vi "GeoData.vi"() -> ()   [LabVIEW 2017] (continued)
48213\tPalestine\tTX\tHenderson County\tH1\n75763\t48213\tFrankston\tTX\tHenderson County\tH1\n75778\t48213\tMurchison\tTX\tHenderson County\tH1\n75751\t48213\tAthens\tTX\tHenderson County\tH1\n75124\t48213\tEustace\tTX\tHenderson County\tH1\n75143\t48213\tKemp\tTX\tHenderson County\tH1\n75782\t48213\tPoynor\tTX\tHenderson County\tH1\n75148\t48213\tMalakoff\tTX\tHenderson County\tH1\n75758\t48213\tChandler\tTX\tHenderson County\tH1\n75147\t48213\tMabank\tTX\tHenderson County\tH1\n75163\t48213\tTrinidad\tTX\tHenderson County\tH1\n75752\t48213\tAthens\tTX\tHenderson County\tH1\n75770\t48213\tLarue\tTX\tHenderson County\tH1\n75756\t48213\tBrownsboro\tTX\tHenderson County\tH1\n75156\t48213\tMabank\tTX\tHenderson County\tH1\n78537\t48215\tDonna\tTX\tHidalgo County\tH1\n78573\t48215\tMission\tTX\tHidalgo County\tH1\n78569\t48215\tLyford\tTX\tHidalgo County\tH1\n78563\t48215\tLinn\tTX\tHidalgo County\tH1\n78502\t48215\tMcallen\tTX\tHidalgo County\tH1\n78501\t48215\tMcallen\tTX\tHidalgo County\tH1\n78599\t48215\tWeslaco\tTX\tHidalgo County\tH1\n78549\t48215\tHargill\tTX\tHidalgo County\tH1\n78504\t48215\tMcallen\tTX\tHidalgo County\tH1\n78516\t48215\tAlamo\tTX\tHidalgo County\tH1\n78538\t48215\tEdcouch\tTX\tHidalgo County\tH1\n78596\t48215\tWeslaco\tTX\tHidalgo County\tH1\n78505\t48215\tMcallen\tTX\tHidalgo County\tH1\n78548\t48215\tGrulla\tTX\tHidalgo County\tH1\n78562\t48215\tLa villa\tTX\tHidalgo County\tH1\n78540\t48215\tEdinburg\tTX\tHidalgo County\tH1\n78558\t48215\tLa blanca\tTX\tHidalgo County\tH1\n78577\t48215\tPharr\tTX\tHidalgo County\tH1\n78570\t48215\tMercedes\tTX\tHidalgo County\tH1\n78579\t48215\tProgreso\tTX\tHidalgo County\tH1\n78595\t48215\tSullivan city\tTX\tHidalgo County\tH1\n78503\t48215\tMcallen\tTX\tHidalgo County\tH1\n78541\t48215\tEdinburg\tTX\tHidalgo County\tH1\n78572\t48215\tMission\tTX\tHidalgo County\tH1\n78557\t48215\tHidalgo\tTX\tHidalgo County\tH1\n78559\t48215\tLa feria\tTX\tHidalgo County\tH1\n78539\t48215\tEdinburg\tTX\tHidalgo County\tH1\n78542\t48215\tEdinburg\tTX\tHidalgo County\tH1\n78574\t48215\tMission\tTX\tHidalgo County\tH1\n78576\t48215\tPenitas\tTX\tHidalgo County\tH1\n78589\t48215\tSan juan\tTX\tHidalgo County\tH1\n78560\t48215\tLa joya\tTX\tHidalgo County\tH1\n78543\t48215\tElsa\tTX\tHidalgo County\tH1\n78565\t48215\tLos ebanos\tTX\tHidalgo County\tH1\n76055\t48217\tItasca\tTX\tHill County\tH1\n76692\t48217\tWhitney\tTX\tHill County\tH1\n76627\t48217\tBlum\tTX\tHill County\tH1\n76622\t48217\tAquilla\tTX\tHill County\tH1\n76093\t48217\tRio vista\tTX\tHill County\tH1\n76676\t48217\tPenelope\tTX\tHill County\tH1\n76628\t48217\tBrandon\tTX\tHill County\tH1\n76621\t48217\tAbbott\tTX\tHill County\tH1\n76631\t48217\tBynum\tTX\tHill County\tH1\n76650\t48217\tIrene\tTX\tHill County\tH1\n76050\t48217\tGrandview\tTX\tHill County\tH1\n76691\t48217\tWest\tTX\tHill County\tH1\n76648\t48217\tHubbard\tTX\tHill County\tH1\n76636\t48217\tCovington\tTX\tHill County\tH1\n76670\t48217\tMilford\tTX\tHill County\tH1\n76645\t48217\tHillsboro\tTX\tHill County\tH1\n76673\t48217\tMount calm\tTX\tHill County\tH1\n76660\t48217\tMalone\tTX\tHill County\tH1\n76666\t48217\tMertens\tTX\tHill County\tH1\n79358\t48219\tRopesville\tTX\tHockley County\tH1\n79407\t48219\tLubbock\tTX\tHockley County\tH1\n79363\t48219\tShallowater\tTX\tHockley County\tH1\n79313\t48219\tAnton\tTX\tHockley County\tH1\n79372\t48219\tSundown\tTX\tHockley County\tH1\n79345\t48219\tMeadow\tTX\tHockley County\tH1\n79367\t48219\tSmyer\tTX\tHockley County\tH1\n79380\t48219\tWhitharral\tTX\tHockley County\tH1\n79339\t48219\tLittlefield\tTX\tHockley County\tH1\n79336\t48219\tLevelland\tTX\tHockley County\tH1\n79353\t48219\tPep\tTX\tHockley County\tH1\n76035\t48221\tCresson\tTX\tHood County\tH1\n76462\t48221\tLipan\tTX\tHood County\tH1\n76048\t48221\tGranbury\tTX\tHood County\tH1\n76033\t48221\tCleburne\tTX\tHood County\tH1\n76049\t48221\tGranbury\tTX\tHood County\tH1\n76433\t48221\tBluff dale\tTX\tHood County\tH1\n76476\t48221\tTolar\tTX\tHood County\tH1\n76087\t48221\tWeatherford\tTX\tHood County\tH1\n76044\t48221\tGodley\tTX\tHood County\tH1\n76467\t48221\tPaluxy\tTX\tHood County\tH1\n75431\t48223\tComo\tTX\tHopkins County\tH1\n75457\t48223\tMount vernon\tTX\tHopkins County\tH1\n75420\t48223\tBrashear\tTX\tHopkins County\tH1\n75497\t48223\tYantis\tTX\tHopkins County\tH1\n75481\t48223\tSulphur bluff\tTX\tHopkins County\tH1\n75453\t48223\tLone oak\tTX\tHopkins County\tH1\n75494\t48223\tWinnsboro\tTX\tHopkins County\tH1\n75437\t48223\tDike\tTX\tHopkins County\tH1\n75482\t48223\tSulphur springs\tTX\tHopkins County\tH1\n75471\t48223\tPickton\tTX\tHopkins County\tH1\n75483\t48223\tSulphur springs\tTX\tHopkins County\tH1\n75433\t48223\tCumby\tTX\tHopkins County\tH1\n75478\t48223\tSaltillo\tTX\tHopkins County\tH1\n75862\t48225\tTrinity\tTX\tHouston County\tH1\n75844\t48225\tGrapeland\tTX\tHouston County\tH1\n75849\t48225\tLatexo\tTX\tHouston County\tH1\n75847\t48225\tKennard\tTX\tHouston County\tH1\n75839\t48225\tElkhart\tTX\tHouston County\tH1\n75858\t48225\tRatcliff\tTX\tHouston County\tH1\n75851\t48225\tLovelady\tTX\tHouston County\tH1\n75835\t48225\tCrockett\tTX\tHouston County\tH1\n79511\t48227\tCoahoma\tTX\tHoward County\tH1\n79720\t48227\tBig spring\tTX\tHoward County\tH1\n79733\t48227\tForsan\tTX\tHoward County\tH1\n79748\t48227\tKnott\tTX\tHoward County\tH1\n79851\t48229\tSierra blanca\tTX\tHudspeth County\tH1\n79837\t48229\tDell city\tTX\tHudspeth County\tH1\n79839\t48229\tFort hancock\tTX\tHudspeth County\tH1\n79938\t48229\tEl paso\tTX\tHudspeth County\tH1\n75474\t48231\tQuinlan\tTX\tHunt County\tH1\n75469\t48231\tPecan gap\tTX\tHunt County\tH1\n75402\t48231\tGreenville\tTX\tHunt County\tH1\n75423\t48231\tCeleste\tTX\tHunt County\tH1\n75169\t48231\tWills point\tTX\tHunt County\tH1\n75442\t48231\tFarmersville\tTX\tHunt County\tH1\n75428\t48231\tCommerce\tTX\tHunt County\tH1\n75422\t48231\tCampbell\tTX\tHunt County\tH1\n75160\t48231\tTerrell\tTX\tHunt County\tH1\n75448\t48231\tKlondike\tTX\tHunt County\tH1\n75401\t48231\tGreenville\tTX\tHunt County\tH1\n75453\t48231\tLone oak\tTX\tHunt County\tH1\n75403\t48231\tGreenville\tTX\tHunt County\tH1\n75496\t48231\tWolfe city\tTX\tHunt County\tH1\n75135\t48231\tCaddo mills\tTX\tHunt County\tH1\n75452\t48231\tLeonard\tTX\tHunt County\tH1\n75449\t48231\tLadonia\tTX\tHunt County\tH1\n75458\t48231\tMerit\tTX\tHunt County\tH1\n75189\t48231\tRoyse city\tTX\tHunt County\tH1\n75404\t48231\tGreenville\tTX\tHunt County\tH1\n79080\t48233\tSkellytown\tTX\tHutchinson County\tH1\n79078\t48233\tSanford\tTX\tHutchinson County\tH1\n79036\t48233\tFritch\tTX\tHutchinson County\tH1\n79008\t48233\tBorger\tTX\tHutchinson County\tH1\n79062\t48233\tMorse\tTX\tHutchinson County\tH1\n79081\t48233\tSpearman\tTX\tHutchinson County\tH1\n79083\t48233\tStinnett\tTX\tHutchinson County\tH1\n79007\t48233\tBorger\tTX\tHutchinson County\tH1\n76941\t48235\tMertzon\tTX\tIrion County\tH1\n76904\t48235\tSan angelo\tTX\tIrion County\tH1\n76901\t48235\tSan angelo\tTX\tIrion County\tH1\n76930\t48235\tBarnhart\tTX\tIrion County\tH1\n76449\t48237\tGraford\tTX\tJack County\tH1\n76459\t48237\tJermyn\tTX\tJack County\tH1\n76487\t48237\tPoolville\tTX\tJack County\tH1\n76486\t48237\tPerrin\tTX\tJack County\tH1\n76426\t48237\tBridgeport\tTX\tJack County\tH1\n76365\t48237\tHenrietta\tTX\tJack County\tH1\n76431\t48237\tChico\tTX\tJack County\tH1\n76427\t48237\tBryson\tTX\tJack County\tH1\n76230\t48237\tBowie\tTX\tJack County\tH1\n76389\t48237\tWindthorst\tTX\tJack County\tH1\n76458\t48237\tJacksboro\tTX\tJack County\tH1\n77979\t48239\tPort lavaca\tTX\tJackson County\tH1\n77957\t48239\tEdna\tTX\tJackson County\tH1\n77465\t48239\tPalacios\tTX\tJackson County\tH1\n77971\t48239\tLolita\tTX\tJackson County\tH1\n77969\t48239\tLa salle\tTX\tJackson County\tH1\n77962\t48239\tGanado\tTX\tJackson County\tH1\n77991\t48239\tVanderbilt\tTX\tJackson County\tH1\n77961\t48239\tFrancitas\tTX\tJackson County\tH1\n77970\t48239\tLa ward\tTX\tJackson County\tH1\n75933\t48241\tCall\tTX\tJasper County\tH1\n75966\t48241\tNewton\tTX\tJasper County\tH1\n77662\t48241\tVidor\tTX\tJasper County\tH1\n75931\t48241\tBrookeland\tTX\tJasper County\tH1\n75951\t48241\tJasper\tTX\tJasper County\tH1\n75980\t48241\tZavalla\tTX\tJasper County\tH1\n75956\t48241\tKirbyville\tTX\tJasper County\tH1\n77615\t48241\tEvadale\tTX\tJasper County\tH1\n77612\t48241\tBuna\tTX\tJasper County\tH1\n79734\t48243\tFort davis\tTX\tJeff Davis County\tH1\n79854\t48243\tValentine\tTX\tJeff Davis County\tH1\n77702\t48245\tBeaumont\tTX\tJefferson County\tH1\n77622\t48245\tHamshire\tTX\tJefferson County\tH1\n77726\t48245\tBeaumont\tTX\tJefferson County\tH1\n77707\t48245\tBeaumont\tTX\tJefferson County\tH1\n77705\t48245\tBeaumont\tTX\tJefferson County\tH1\n77651\t48245\tPort neches\tTX\tJefferson County\tH1\n77613\t48245\tChina\tTX\tJefferson County\tH1\n77665\t48245\tWinnie\tTX\tJefferson County\tH1\n77619\t48245\tGroves\tTX\tJefferson County\tH1\n77655\t48245\tSabine pass\tTX\tJefferson County\tH1\n77629\t48245\tNome\tTX\tJefferson County\tH1\n77706\t48245\tBeaumont\tTX\tJefferson County\tH1\n77720\t48245\tBeaumont\tTX\tJefferson County\tH1\n77725\t48245\tBeaumont\tTX\tJefferson County\tH1\n77642\t48245\tPort arthur\tTX\tJefferson County\tH1\n77657\t48245\tLumberton\tTX\tJefferson County\tH1\n77701\t48245\tBeaumont\tTX\tJefferson County\tH1\n77704\t48245\tBeaumont\tTX\tJefferson County\tH1\n77708\t48245\tBeaumont\tTX\tJefferson County\tH1\n77713\t48245\tBeaumont\tTX\tJefferson County\tH1\n77627\t48245\tNederland\tTX\tJefferson County\tH1\n77640\t48245\tPort arthur\tTX\tJefferson County\tH1\n77703\t48245\tBeaumont\tTX\tJefferson County\tH1\n78582\t48247\tRio grande city\tTX\tJim Hogg County\tH1\n78360\t48247\tGuerra\tTX\tJim Hogg County\tH1\n78361\t48247\tHebbronville\tTX\tJim Hogg County\tH1\n78383\t48249\tSandia\tTX\tJim Wells County\tH1\n78372\t48249\tOrange grove\tTX\tJim Wells County\tH1\n78375\t48249\tPremont\tTX\tJim Wells County\tH1\n78384\t48249\tSan diego\tTX\tJim Wells County\tH1\n78342\t48249\tBen bolt\tTX\tJim Wells County\tH1\n78332\t48249\tAlice\tTX\tJim Wells County\tH1\n78380\t48249\tRobstown\tTX\tJim Wells County\tH1\n76059\t48251\tKeene\tTX\tJohnson County\tH1\n76035\t48251\tCresson\tTX\tJohnson County\tH1\n76084\t48251\tVenus\tTX\tJohnson County\tH1\n76033\t48251\tCleburne\tTX\tJohnson County\tH1\n76093\t48251\tRio vista\tTX\tJohnson County\tH1\n76009\t48251\tAlvarado\tTX\tJohnson County\tH1\n76061\t48251\tLillian\tTX\tJohnson County\tH1\n76058\t48251\tJoshua\tTX\tJohnson County\tH1\n76049\t48251\tGranbury\tTX\tJohnson County\tH1\n76050\t48251\tGrandview\tTX\tJohnson County\tH1\n76036\t48251\tCrowley\tTX\tJohnson County\tH1\n76097\t48251\tBurleson\tTX\tJohnson County\tH1\n76031\t48251\tCleburne\tTX\tJohnson County\tH1\n76063\t48251\tMansfield\tTX\tJohnson County\tH1\n76028\t48251\tBurleson\tTX\tJohnson County\tH1\n76044\t48251\tGodley\tTX\tJohnson County\tH1\n76070\t48251\tNemo\tTX\tJohnson County\tH1\n79536\t48253\tMerkel\tTX\tJones County\tH1\n79521\t48253\tHaskell\tTX\tJones County\tH1\n79520\t48253\tHamlin\tTX\tJones County\tH1\n79553\t48253\tStamford\tTX\tJones County\tH1\n79525\t48253\tHawley\tTX\tJones County\tH1\n79503\t48253\tAvoca\tTX\tJones County\tH1\n79501\t48253\tAnson\tTX\tJones County\tH1\n79601\t48253\tAbilene\tTX\tJones County\tH1\n79561\t48253\tTrent\tTX\tJones County\tH1\n79560\t48253\tSylvester\tTX\tJones County\tH1\n79533\t48253\tLueders\tTX\tJones County\tH1\n78113\t48255\tFalls city\tTX\tKarnes County\tH1\n78117\t48255\tHobson\tTX\tKarnes County\tH1\n78111\t48255\tEcleto\tTX\tKarnes County\tH1\n78119\t48255\tKenedy\tTX\tKarnes County\tH1\n78116\t48255\tGillett\tTX\tKarnes County\tH1\n78118\t48255\tKarnes city\tTX\tKarnes County\tH1\n78144\t48255\tPanna maria\tTX\tKarnes County\tH1\n78151\t48255\tRunge\tTX\tKarnes County\tH1\n78062\t48255\tPeggy\tTX\tKarnes County\tH1\n75114\t48257\tCrandall\tTX\tKaufman County\tH1\n75142\t48257\tKaufman\tTX\tKaufman County\tH1\n75474\t48257\tQuinlan\tTX\tKaufman County\tH1\n75159\t48257\tSeagoville\tTX\tKaufman County\tH1\n75157\t48257\tRosser\tTX\tKaufman County\tH1\n75032\t48257\tRockwall\tTX\tKaufman County\tH1\n75158\t48257\tScurry\tTX\tKaufman County\tH1\n75169\t48257\tWills point\tTX\tKaufman County\tH1\n75118\t48257\tElmo\tTX\tKaufman County\tH1\n75143\t48257\tKemp\tTX\tKaufman County\tH1\n75161\t48257\tTerrell\tTX\tKaufman County\tH1\n75160\t48257\tTerrell\tTX\tKaufman County\tH1\n75147\t48257\tMabank\tTX\tKaufman County\tH1\n75182\t48257\tSunnyvale\tTX\tKaufman County\tH1\n75126\t48257\tForney\tTX\tKaufman County\tH1\n75156\t48257\tMabank\tTX\tKaufman County\tH1\n78004\t48259\tBergheim\tTX\tKendall County\tH1\n78074\t48259\tWaring\tTX\tKendall County\tH1\n78027\t48259\tKendalia\tTX\tKendall County\tH1\n78006\t48259\tBoerne\tTX\tKendall County\tH1\n78624\t48259\tFredericksburg\tTX\tKendall County\tH1\n78013\t48259\tComfort\tTX\tKendall County\tH1\n78015\t48259\tBoerne\tTX\tKendall County\tH1\n78070\t48259\tSpring branch\tTX\tKendall County\tH1\n78606\t48259\tBlanco\tTX\tKendall County\tH1\n78385\t48261\tSarita\tTX\tKenedy County\tH1\n78338\t48261\tArmstrong\tTX\tKenedy County\tH1\n79528\t48263\tJayton\tTX\tKent County\tH1\n79549\t48263\tSnyder\tTX\tKent County\tH1\n79518\t48263\tGirard\tTX\tKent County\tH1\n78055\t48265\tMedina\tTX\tKerr County\tH1\n76849\t48265\tJunction\tTX\tKerr County\tH1\n78010\t48265\tCenter point\tTX\tKerr County\tH1\n78025\t48265\tIngram\tTX\tKerr County\tH1\n78024\t48265\tHunt\tTX\tKerr County\tH1\n78063\t48265\tPipe creek\tTX\tKerr County\tH1\n78624\t48265\tFredericksburg\tTX\tKerr County\tH1\n78013\t48265\tComfort\tTX\tKerr County\tH1\n78631\t48265\tHarper\tTX\tKerr County\tH1\n78058\t48265\tMountain home\tTX\tKerr County\tH1\n78029\t48265\tKerrville\tTX\tKerr County\tH1\n78028\t48265\tKerrville\tTX\tKerr County\tH1\n78003\t48265\tBandera\tTX\tKerr County\tH1\n76859\t48267\tMenard\tTX\tKimble County\tH1\n76849\t48267\tJunction\tTX\tKimble County\tH1\n76856\t48267\tMason\tTX\tKimble County\tH1\n78631\t48267\tHarper\tTX\tKimble County\tH1\n76883\t48267\tTelegraph\tTX\tKimble County\tH1\n76854\t48267\tLondon\tTX\tKimble County\tH1\n76874\t48267\tRoosevelt\tTX\tKimble County\tH1\n79236\t48269\tGuthrie\tTX\tKing County\tH1\n79248\t48269\tPaducah\tTX\tKing County\tH1\n78832\t48271\tBrackettville\tTX\tKinney County\tH1\n78877\t48271\tQuemado\tTX\tKinney County\tH1\n78363\t48273\tKingsville\tTX\tKleberg County\tH1\n78379\t48273\tRiviera\tTX\tKleberg County\tH1\n79227\t48275\tCrowell\tTX\tKnox County\tH1\n79505\t48275\tBenjamin\tTX\tKnox County\tH1\n76380\t48275\tSeymour\tTX\tKnox County\tH1\n76371\t48275\tMunday\tTX\tKnox County\tH1\n79529\t48275\tKnox city\tTX\tKnox County\tH1\n76363\t48275\tGoree\tTX\tKnox County\tH1\n75421\t48277\tBrookston\tTX\tLamar County\tH1\n75411\t48277\tArthur city\tTX\tLamar County\tH1\n75470\t48277\tPetty\tTX\tLamar County\tH1\n75416\t48277\tBlossom\tTX\tLamar County\tH1\n75461\t48277\tParis\tTX\tLamar County\tH1\n75477\t48277\tRoxton\tTX\tLamar County\tH1\n75462\t48277\tParis\tTX\tLamar County\tH1\n75434\t48277\tCunningham\tTX\tLamar County\tH1\n75435\t48277\tDeport\tTX\tLamar County\tH1\n75436\t48277\tDetroit\tTX\tLamar County\tH1\n75417\t48277\tBogata\tTX\tLamar County\tH1\n75468\t48277\tPattonville\tTX\tLamar County\tH1\n75460\t48277\tParis\tTX\tLamar County\tH1\n75473\t48277\tPowderly\tTX\tLamar County\tH1\n75486\t48277\tSumner\tTX\tLamar County\tH1\n75425\t48277\tChicota\tTX\tLamar County\tH1\n75446\t48277\tHoney grove\tTX\tLamar County\tH1\n79064\t48279\tOlton\tTX\tLamb County\tH1\n79031\t48279\tEarth\tTX\tLamb County\tH1\n79326\t48279\tFieldton\tTX\tLamb County\tH1\n79369\t48279\tSpade\tTX\tLamb County\tH1\n79312\t48279\tAmherst\tTX\tLamb County\tH1\n79313\t48279\tAnton\tTX\tLamb County\tH1\n79347\t48279\tMuleshoe\tTX\tLamb County\tH1\n79082\t48279\tSpringlake\tTX\tLamb County\tH1\n79339\t48279\tLittlefield\tTX\tLamb County\tH1\n79371\t48279\tSudan\tTX\tLamb County\tH1\n76550\t48281\tLampasas\tTX\tLampasas County\tH1\n76528\t48281\tGatesville\tTX\tLampasas County\tH1\n76853\t48281\tLometa\tTX\tLampasas County\tH1\n76539\t48281\tKempner\tTX\tLampasas County\tH1\n76525\t48281\tEvant\tTX\tLampasas County\tH1\n76522\t48281\tCopperas cove\tTX\tLampasas County\tH1\n76824\t48281\tBend\tTX\tLampasas County\tH1\n78001\t48283\tArtesia wells\tTX\tLa Salle County\tH1\n78014\t48283\tCotulla\tTX\tLa Salle County\tH1\n78021\t48283\tFowlerton\tTX\tLa Salle County\tH1\n78019\t48283\tEncinal\tTX\tLa Salle County\tH1\n77986\t48285\tSublime\tTX\tLavaca County\tH1\n77975\t48285\tMoulton\tTX\tLavaca County\tH1\n77987\t48285\tSweet home\tTX\tLavaca County\tH1\n78941\t48285\tFlatonia\tTX\tLavaca County\tH1\n78956\t48285\tSchulenburg\tTX\tLavaca County\tH1\n77984\t48285\tShiner\tTX\tLavaca County\tH1\n78629\t48285\tGonzales\tTX\tLavaca County\tH1\n77995\t48285\tYoakum\tTX\tLavaca County\tH1\n77964\t48285\tHallettsville\tTX\tLavaca County\tH1\n78942\t48287\tGiddings\tTX\tLee County\tH1\n78947\t48287\tLexington\tTX\tLee County\tH1\n76578\t48287\tThrall\tTX\tLee County\tH1\n78659\t48287\tPaige\tTX\tLee County\tH1\n78946\t48287\tLedbetter\tTX\tLee County\tH1\n78650\t48287\tMc dade\tTX\tLee County\tH1\n77853\t48287\tDime box\tTX\tLee County\tH1\n78948\t48287\tLincoln\tTX\tLee County\tH1\n78621\t48287\tElgin\tTX\tLee County\tH1\n78945\t48287\tLa grange\tTX\tLee County\tH1\n75833\t48289\tCenterville\tTX\tLeon County\tH1\n77871\t48289\tNormangee\tTX\tLeon County\tH1\n77865\t48289\tMarquez\tTX\tLeon County\tH1\n75846\t48289\tJewett\tTX\tLeon County\tH1\n75852\t48289\tMidway\tTX\tLeon County\tH1\n75850\t48289\tLeona\tTX\tLeon County\tH1\n75831\t48289\tBuffalo\tTX\tLeon County\tH1\n77864\t48289\tMadisonville\tTX\tLeon County\tH1\n75855\t48289\tOakwood\tTX\tLeon County\tH1\n77855\t48289\tFlynn\tTX\tLeon County\tH1\n77850\t48289\tConcord\tTX\tLeon County\tH1\n77371\t48291\tShepherd\tTX\tLiberty County\tH1\n77597\t48291\tWallisville\tTX\tLiberty County\tH1\n77533\t48291\tDaisetta\tTX\tLiberty County\tH1\n77327\t48291\tCleveland\tTX\tLiberty County\tH1\n77328\t48291\tCleveland\tTX\tLiberty County\tH1\n77535\t48291\tDayton\tTX\tLiberty County\tH1\n77564\t48291\tHull\tTX\tLiberty County\tH1\n77582\t48291\tRaywood\tTX\tLiberty County\tH1\n77561\t48291\tHardin\tTX\tLiberty County\tH1\n77357\t48291\tNew caney\tTX\tLiberty County\tH1\n77369\t48291\tRye\tTX\tLiberty County\tH1\n77575\t48291\tLiberty\tTX\tLiberty County\tH1\n77538\t48291\tDevers\tTX\tLiberty County\tH1\n77372\t48291\tSplendora\tTX\tLiberty County\tH1\n77368\t48291\tRomayor\tTX\tLiberty County\tH1\n75838\t48293\tDonie\tTX\tLimestone County\tH1\n76664\t48293\tMart\tTX\tLimestone County\tH1\n75846\t48293\tJewett\tTX\tLimestone County\tH1\n76624\t48293\tAxtell\tTX\tLimestone County\tH1\n76667\t48293\tMexia\tTX\tLimestone County\tH1\n76686\t48293\tTehuacana\tTX\tLimestone County\tH1\n76653\t48293\tKosse\tTX\tLimestone County\tH1\n76642\t48293\tGroesbeck\tTX\tLimestone County\tH1\n76635\t48293\tCoolidge\tTX\tLimestone County\tH1\n76687\t48293\tThornton\tTX\tLimestone County\tH1\n76693\t48293\tWortham\tTX\tLimestone County\tH1\n76673\t48293\tMount calm\tTX\tLimestone County\tH1\n76678\t48293\tPrairie hill\tTX\tLimestone County\tH1\n79005\t48295\tBooker\tTX\tLipscomb County\tH1\n79034\t48295\tFollett\tTX\tLipscomb County\tH1\n79056\t48295\tLipscomb\tTX\tLipscomb County\tH1\n79024\t48295\tDarrouzett\tTX\tLipscomb County\tH1\n79046\t48295\tHiggins\tTX\tLipscomb County\tH1\n78102\t48297\tBeeville\tTX\tLive Oak County\tH1\n78383\t48297\tSandia\tTX\tLive Oak County\tH1\n78372\t48297\tOrange grove\tTX\tLive Oak County\tH1\n78389\t48297\tSkidmore\tTX\tLive Oak County\tH1\n78075\t48297\tWhitsett\tTX\tLive Oak County\tH1\n78071\t48297\tThree rivers\tTX\tLive Oak County\tH1\n78368\t48297\tMathis\tTX\tLive Oak County\tH1\n78060\t48297\tOakville\tTX\tLive Oak County\tH1\n78008\t48297\tCampbellton\tTX\tLive Oak County\tH1\n78350\t48297\tDinero\tTX\tLive Oak County\tH1\n78022\t48297\tGeorge west\tTX\tLive Oak County\tH1\n76885\t48299\tValley spring\tTX\tLlano County\tH1\n78643\t48299\tLlano\tTX\tLlano County\tH1\n78609\t48299\tBuchanan dam\tTX\tLlano County\tH1\n78639\t48299\tKingsland\tTX\tLlano County\tH1\n78607\t48299\tBluffton\tTX\tLlano County\tH1\n78624\t48299\tFredericksburg\tTX\tLlano County\tH1\n78611\t48299\tBurnet\tTX\tLlano County\tH1\n78657\t48299\tHorseshoe bay\tTX\tLlano County\tH1\n78672\t48299\tTow\tTX\tLlano County\tH1\n76831\t48299\tCastell\tTX\tLlano County\tH1\n79754\t48301\tMentone\tTX\tLoving County\tH1\n79499\t48303\tLubbock\tTX\tLubbock County\tH1\n79358\t48303\tRopesville\tTX\tLubbock County\tH1\n79366\t48303\tRansom canyon\tTX\tLubbock County\tH1\n79350\t48303\tNew deal\tTX\tLubbock County\tH1\n79424\t48303\tLubbock\tTX\tLubbock County\tH1\n79382\t48303\tWolfforth\tTX\tLubbock County\tH1\n79407\t48303\tLubbock\tTX\tLubbock County\tH1\n79453\t48303\tLubbock\tTX\tLubbock County\tH1\n79409\t48303\tLubbock\tTX\tLubbock County\tH1\n79402\t48303\tLubbock\tTX\tLubbock County\tH1\n79404\t48303\tLubbock\tTX\tLubbock County\tH1\n79412\t48303\tLubbock\tTX\tLubbock County\tH1\n79410\t48303\tLubbock\tTX\tLubbock County\tH1\n79343\t48303\tLorenzo\tTX\tLubbock County\tH1\n79430\t48303\tLubbock\tTX\tLubbock County\tH1\n79381\t48303\tWilson\tTX\tLubbock County\tH1\n79329\t48303\tIdalou\tTX\tLubbock County\tH1\n79415\t48303\tLubbock\tTX\tLubbock County\tH1\n79416\t48303\tLubbock\tTX\tLubbock County\tH1\n79411\t48303\tLubbock\tTX\tLubbock County\tH1\n79493\t48303\tLubbock\tTX\tLubbock County\tH1\n79464\t48303\tLubbock\tTX\tLubbock County\tH1\n79406\t48303\tLubbock\tTX\tLubbock County\tH1\n79373\t48303\tTahoka\tTX\tLubbock County\tH1\n79401\t48303\tLubbock\tTX\tLubbock County\tH1\n79363\t48303\tShallowater\tTX\tLubbock County\tH1\n79313\t48303\tAnton\tTX\tLubbock County\tH1\n79490\t48303\tLubbock\tTX\tLubbock County\tH1\n79491\t48303\tLubbock\tTX\tLubbock County\tH1\n79311\t48303\tAbernathy\tTX\tLubbock County\tH1\n79364\t48303\tSlaton\tTX\tLubbock County\tH1\n79408\t48303\tLubbock\tTX\tLubbock County\tH1\n79403\t48303\tLubbock\tTX\tLubbock County\tH1\n79413\t48303\tLubbock\tTX\tLubbock County\tH1\n79423\t48303\tLubbock\tTX\tLubbock County\tH1\n79414\t48303\tLubbock\tTX\tLubbock County\tH1\n79452\t48303\tLubbock\tTX\tLubbock County\tH1\n79356\t48305\tPost\tTX\tLynn County\tH1\n79331\t48305\tLamesa\tTX\tLynn County\tH1\n79381\t48305\tWilson\tTX\tLynn County\tH1\n79373\t48305\tTahoka\tTX\tLynn County\tH1\n79351\t48305\tOdonnell\tTX\tLynn County\tH1\n79364\t48305\tSlaton\tTX\tLynn County\tH1\n79345\t48305\tMeadow\tTX\tLynn County\tH1\n79423\t48305\tLubbock\tTX\tLynn County\tH1\n79383\t48305\tNew home\tTX\tLynn County\tH1\n76852\t48307\tLohn\tTX\tMcCulloch County\tH1\n76872\t48307\tRochelle\tTX\tMcCulloch County\tH1\n76825\t48307\tBrady\tTX\tMcCulloch County\tH1\n76858\t48307\tMelvin\tTX\tMcCulloch County\tH1\n76836\t48307\tDoole\tTX\tMcCulloch County\tH1\n76887\t48307\tVoca\tTX\tMcCulloch County\tH1\n76705\t48309\tWaco\tTX\tMcLennan County\tH1\n76633\t48309\tChina spring\tTX\tMcLennan County\tH1\n76664\t48309\tMart\tTX\tMcLennan County\tH1\n76704\t48309\tWaco\tTX\tMcLennan County\tH1\n76557\t48309\tMoody\tTX\tMcLennan County\tH1\n76655\t48309\tLorena\tTX\tMcLennan County\tH1\n76622\t48309\tAquilla\tTX\tMcLennan County\tH1\n76684\t48309\tRoss\tTX\tMcLennan County\tH1\n76797\t48309\tWaco\tTX\tMcLennan County\tH1\n76711\t48309\tWaco\tTX\tMcLennan County\tH1\n76703\t48309\tWaco\tTX\tMcLennan County\tH1\n76630\t48309\tBruceville\tTX\tMcLennan County\tH1\n76640\t48309\tElm mott\tTX\tMcLennan County\tH1\n76621\t48309\tAbbott\tTX\tMcLennan County\tH1\n76716\t48309\tWaco\tTX\tMcLennan County\tH1\n76708\t48309\tWaco\tTX\tMcLennan County\tH1\n76682\t48309\tRiesel\tTX\tMcLennan County\tH1\n76624\t48309\tAxtell\tTX\tMcLennan County\tH1\n76710\t48309\tWaco\tTX\tMcLennan County\tH1\n76689\t48309\tValley mills\tTX\tMcLennan County\tH1\n76706\t48309\tWaco\tTX\tMcLennan County\tH1\n76707\t48309\tWaco\tTX\tMcLennan County\tH1\n76643\t48309\tHewitt\tTX\tMcLennan County\tH1\n76657\t48309\tMc gregor\tTX\tMcLennan County\tH1\n76638\t48309\tCrawford\tTX\tMcLennan County\tH1\n76702\t48309\tWaco\tTX\tMcLennan County\tH1\n76798\t48309\tWaco\tTX\tMcLennan County\tH1\n76691\t48309\tWest\tTX\tMcLennan County\tH1\n76701\t48309\tWaco\tTX\tMcLennan County\tH1\n76561\t48309\tOglesby\tTX\tMcLennan County\tH1\n76712\t48309\tWoodway\tTX\tMcLennan County\tH1\n76524\t48309\tEddy\tTX\tMcLennan County\tH1\n76714\t48309\tWaco\tTX\tMcLennan County\tH1\n76799\t48309\tWaco\tTX\tMcLennan County\tH1\n76673\t48309\tMount calm\tTX\tMcLennan County\tH1\n76654\t48309\tLeroy\tTX\tMcLennan County\tH1\n78071\t48311\tThree rivers\tTX\tMcMullen County\tH1\n78007\t48311\tCalliham\tTX\tMcMullen County\tH1\n78072\t48311\tTilden\tTX\tMcMullen County\tH1\n78026\t48311\tJourdanton\tTX\tMcMullen County\tH1\n77871\t48313\tNormangee\tTX\tMadison County\tH1\n75852\t48313\tMidway\tTX\tMadison County\tH1\n77872\t48313\tNorth zulch\tTX\tMadison County\tH1\n77861\t48313\tIola\tTX\tMadison County\tH1\n77864\t48313\tMadisonville\tTX\tMadison County\tH1\n77831\t48313\tBedias\tTX\tMadison County\tH1\n75630\t48315\tAvinger\tTX\tMarion County\tH1\n75555\t48315\tBivins\tTX\tMarion County\tH1\n75564\t48315\tLodi\tTX\tMarion County\tH1\n75657\t48315\tJefferson\tTX\tMarion County\tH1\n75683\t48315\tOre city\tTX\tMarion County\tH1\n75651\t48315\tHarleton\tTX\tMarion County\tH1\n75640\t48315\tDiana\tTX\tMarion County\tH1\n75668\t48315\tLone star\tTX\tMarion County\tH1\n79782\t48317\tStanton\tTX\tMartin County\tH1\n79783\t48317\tTarzan\tTX\tMartin County\tH1\n79331\t48317\tLamesa\tTX\tMartin County\tH1\n79749\t48317\tLenorah\tTX\tMartin County\tH1\n79705\t48317\tMidland\tTX\tMartin County\tH1\n76869\t48319\tPontotoc\tTX\tMason County\tH1\n76825\t48319\tBrady\tTX\tMason County\tH1\n78624\t48319\tFredericksburg\tTX\tMason County\tH1\n76856\t48319\tMason\tTX\tMason County\tH1\n76842\t48319\tFredonia\tTX\tMason County\tH1\n76831\t48319\tCastell\tTX\tMason County\tH1\n76820\t48319\tArt\tTX\tMason County\tH1\n77422\t48321\tBrazoria\tTX\tMatagorda County\tH1\n77465\t48321\tPalacios\tTX\tMatagorda County\tH1\n77414\t48321\tBay city\tTX\tMatagorda County\tH1\n77404\t48321\tBay city\tTX\tMatagorda County\tH1\n77456\t48321\tMarkham\tTX\tMatagorda County\tH1\n77420\t48321\tBoling\tTX\tMatagorda County\tH1\n77457\t48321\tMatagorda\tTX\tMatagorda County\tH1\n77428\t48321\tCollegeport\tTX\tMatagorda County\tH1\n77482\t48321\tVan vleck\tTX\tMatagorda County\tH1\n77458\t48321\tMidfield\tTX\tMatagorda County\tH1\n77415\t48321\tCedar lane\tTX\tMatagorda County\tH1\n77480\t48321\tSweeny\tTX\tMatagorda County\tH1\n77468\t48321\tPledger\tTX\tMatagorda County\tH1\n77419\t48321\tBlessing\tTX\tMatagorda County\tH1\n77440\t48321\tElmaton\tTX\tMatagorda County\tH1\n77483\t48321\tWadsworth\tTX\tMatagorda County\tH1\n78852\t48323\tEagle pass\tTX\tMaverick County\tH1\n78860\t48323\tEl indio\tTX\tMaverick County\tH1\n78853\t48323\tEagle pass\tTX\tMaverick County\tH1\n78877\t48323\tQuemado\tTX\tMaverick County\tH1\n78023\t48325\tHelotes\tTX\tMedina County\tH1\n78039\t48325\tLa coste\tTX\tMedina County\tH1\n78861\t48325\tHondo\tTX\tMedina County\tH1\n78886\t48325\tYancey\tTX\tMedina County\tH1\n78056\t48325\tMico\tTX\tMedina County\tH1\n78066\t48325\tRio medina\tTX\tMedina County\tH1\n78016\t48325\tDevine\tTX\tMedina County\tH1\n78057\t48325\tMoore\tTX\tMedina County\tH1\n78052\t48325\tLytle\tTX\tMedina County\tH1\n78253\t48325\tSan antonio\tTX\tMedina County\tH1\n78254\t48325\tSan antonio\tTX\tMedina County\tH1\n78884\t48325\tUtopia\tTX\tMedina County\tH1\n78850\t48325\tD hanis\tTX\tMedina County\tH1\n78009\t48325\tCastroville\tTX\tMedina County\tH1\n78059\t48325\tNatalia\tTX\tMedina County\tH1\n78003\t48325\tBandera\tTX\tMedina County\tH1\n76859\t48327\tMenard\tTX\tMenard County\tH1\n76849\t48327\tJunction\tTX\tMenard County\tH1\n76841\t48327\tFort mc kavett\tTX\tMenard County\tH1\n76825\t48327\tBrady\tTX\tMenard County\tH1\n76848\t48327\tHext\tTX\tMenard County\tH1\n76854\t48327\tLondon\tTX\tMenard County\tH1\n79708\t48329\tMidland\tTX\tMidland County\tH1\n79782\t48329\tStanton\tTX\tMidland County\tH1\n79707\t48329\tMidland\tTX\tMidland County\tH1\n79763\t48329\tOdessa\tTX\tMidland County\tH1\n79765\t48329\tOdessa\tTX\tMidland County\tH1\n79706\t48329\tMidland\tTX\tMidland County\tH1\n79702\t48329\tMidland\tTX\tMidland County\tH1\n79704\t48329\tMidland\tTX\tMidland County\tH1\n79705\t48329\tMidland\tTX\tMidland County\tH1\n79703\t48329\tMidland\tTX\tMidland County\tH1\n79710\t48329\tMidland\tTX\tMidland County\tH1\n79712\t48329\tMidland\tTX\tMidland County\tH1\n79766\t48329\tOdessa\tTX\tMidland County\tH1\n79701\t48329\tMidland\tTX\tMidland County\tH1\n79711\t48329\tMidland\tTX\tMidland County\tH1\n76569\t48331\tRogers\tTX\tMilam County\tH1\n76519\t48331\tBurlington\tTX\tMilam County\tH1\n76523\t48331\tDavilla\tTX\tMilam County\tH1\n76577\t48331\tThorndale\tTX\tMilam County\tH1\n76578\t48331\tThrall\tTX\tMilam County\tH1\n76520\t48331\tCameron\tTX\tMilam County\tH1\n76556\t48331\tMilano\tTX\tMilam County\tH1\n76567\t48331\tRockdale\tTX\tMilam County\tH1\n76530\t48331\tGranger\tTX\tMilam County\tH1\n76570\t48331\tRosebud\tTX\tMilam County\tH1\n77857\t48331\tGause\tTX\tMilam County\tH1\n76518\t48331\tBuckholts\tTX\tMilam County\tH1\n76511\t48331\tBartlett\tTX\tMilam County\tH1\n76534\t48331\tHolland\tTX\tMilam County\tH1\n76864\t48333\tMullin\tTX\tMills County\tH1\n76890\t48333\tZephyr\tTX\tMills County\tH1\n76442\t48333\tComanche\tTX\tMills County\tH1\n76844\t48333\tGoldthwaite\tTX\tMills County\tH1\n76870\t48333\tPriddy\tTX\tMills County\tH1\n76880\t48333\tStar\tTX\tMills County\tH1\n79512\t48335\tColorado city\tTX\tMitchell County\tH1\n79532\t48335\tLoraine\tTX\tMitchell County\tH1\n79545\t48335\tRoscoe\tTX\tMitchell County\tH1\n79565\t48335\tWestbrook\tTX\tMitchell County\tH1\n76225\t48337\tAlvord\tTX\tMontague County\tH1\n76252\t48337\tMuenster\tTX\tMontague County\tH1\n76265\t48337\tSaint jo\tTX\tMontague County\tH1\n76251\t48337\tMontague\tTX\tMontague County\tH1\n76234\t48337\tDecatur\tTX\tMontague County\tH1\n76255\t48337\tNocona\tTX\tMontague County\tH1\n76228\t48337\tBellevue\tTX\tMontague County\tH1\n76270\t48337\tSunset\tTX\tMontague County\tH1\n76239\t48337\tForestburg\tTX\tMontague County\tH1\n76230\t48337\tBowie\tTX\tMontague County\tH1\n76261\t48337\tRinggold\tTX\tMontague County\tH1\n77381\t48339\tSpring\tTX\tMontgomery County\tH1\n77355\t48339\tMagnolia\tTX\tMontgomery County\tH1\n77358\t48339\tNew waverly\tTX\tMontgomery County\tH1\n77389\t48339\tSpring\tTX\tMontgomery County\tH1\n77387\t48339\tSpring\tTX\tMontgomery County\tH1\n77303\t48339\tConroe\tTX\tMontgomery County\tH1\n77356\t48339\tMontgomery\tTX\tMontgomery County\tH1\n77362\t48339\tPinehurst\tTX\tMontgomery County\tH1\n77327\t48339\tCleveland\tTX\tMontgomery County\tH1\n77328\t48339\tCleveland\tTX\tMontgomery County\tH1\n77306\t48339\tConroe\tTX\tMontgomery County\tH1\n77378\t48339\tWillis\tTX\tMontgomery County\tH1\n77353\t48339\tMagnolia\tTX\tMontgomery County\tH1\n77339\t48339\tKingwood\tTX\tMontgomery County\tH1\n77301\t48339\tConroe\tTX\tMontgomery County\tH1\n77318\t48339\tWillis\tTX\tMontgomery County\tH1\n77302\t48339\tConroe\tTX\tMontgomery County\tH1\n77379\t48339\tSpring\tTX\tMontgomery County\tH1\n77385\t48339\tConroe\tTX\tMontgomery County\tH1\n77384\t48339\tConroe\tTX\tMontgomery County\tH1\n77447\t48339\tHockley\tTX\tMontgomery County\tH1\n77333\t48339\tDobbin\tTX\tMontgomery County\tH1\n77357\t48339\tNew caney\tTX\tMontgomery County\tH1\n77365\t48339\tPorter\tTX\tMontgomery County\tH1\n77304\t48339\tConroe\tTX\tMontgomery County\tH1\n77386\t48339\tSpring\tTX\tMontgomery County\tH1\n77382\t48339\tSpring\tTX\tMontgomery County\tH1\n77873\t48339\tRichards\tTX\tMontgomery County\tH1\n77354\t48339\tMagnolia\tTX\tMontgomery County\tH1\n77316\t48339\tMontgomery\tTX\tMontgomery County\tH1\n77305\t48339\tConroe\tTX\tMontgomery County\tH1\n77380\t48339\tSpring\tTX\tMontgomery County\tH1\n77372\t48339\tSplendora\tTX\tMontgomery County\tH1\n77393\t48339\tSpring\tTX\tMontgomery County\tH1\n79018\t48341\tChanning\tTX\tMoore County\tH1\n79029\t48341\tDumas\tTX\tMoore County\tH1\n79036\t48341\tFritch\tTX\tMoore County\tH1\n79083\t48341\tStinnett\tTX\tMoore County\tH1\n79058\t48341\tMasterson\tTX\tMoore County\tH1\n79086\t48341\tSunray\tTX\tMoore County\tH1\n79013\t48341\tCactus\tTX\tMoore County\tH1\n75638\t48343\tDaingerfield\tTX\tMorris County\tH1\n75636\t48343\tCason\tTX\tMorris County\tH1\n75558\t48343\tCookville\tTX\tMorris County\tH1\n75568\t48343\tNaples\tTX\tMorris County\tH1\n75571\t48343\tOmaha\tTX\tMorris County\tH1\n75656\t48343\tHughes springs\tTX\tMorris County\tH1\n75668\t48343\tLone star\tTX\tMorris County\tH1\n79256\t48345\tRoaring springs\tTX\tMotley County\tH1\n79241\t48345\tLockney\tTX\tMotley County\tH1\n79255\t48345\tQuitaque\tTX\tMotley County\tH1\n79235\t48345\tFloydada\tTX\tMotley County\tH1\n79244\t48345\tMatador\tTX\tMotley County\tH1\n79234\t48345\tFlomot\tTX\tMotley County\tH1\n75788\t48347\tSacul\tTX\tNacogdoches County\tH1\n75760\t48347\tCushing\tTX\tNacogdoches County\tH1\n75944\t48347\tEtoile\tTX\tNacogdoches County\tH1\n75961\t48347\tNacogdoches\tTX\tNacogdoches County\tH1\n75964\t48347\tNacogdoches\tTX\tNacogdoches County\tH1\n75965\t48347\tNacogdoches\tTX\tNacogdoches County\tH1\n75943\t48347\tDouglass\tTX\tNacogdoches County\tH1\n75963\t48347\tNacogdoches\tTX\tNacogdoches County\tH1\n75958\t48347\tMartinsville\tTX\tNacogdoches County\tH1\n75937\t48347\tChireno\tTX\tNacogdoches County\tH1\n75946\t48347\tGarrison\tTX\tNacogdoches County\tH1\n75978\t48347\tWoden\tTX\tNacogdoches County\tH1\n75109\t48349\tCorsicana\tTX\tNavarro County\tH1\n75859\t48349\tStreetman\tTX\tNavarro County\tH1\n76679\t48349\tPurdon\tTX\tNavarro County\tH1\n75151\t48349\tCorsicana\tTX\tNavarro County\tH1\n75110\t48349\tCorsicana\tTX\tNavarro County\tH1\n75105\t48349\tChatfield\tTX\tNavarro County\tH1\n76641\t48349\tFrost\tTX\tNavarro County\tH1\n75153\t48349\tPowell\tTX\tNavarro County\tH1\n76626\t48349\tBlooming grove\tTX\tNavarro County\tH1\n75119\t48349\tEnnis\tTX\tNavarro County\tH1\n75102\t48349\tBarry\tTX\tNavarro County\tH1\n76648\t48349\tHubbard\tTX\tNavarro County\tH1\n76681\t48349\tRichland\tTX\tNavarro County\tH1\n75144\t48349\tKerens\tTX\tNavarro County\tH1\n76670\t48349\tMilford\tTX\tNavarro County\tH1\n76639\t48349\tDawson\tTX\tNavarro County\tH1\n75155\t48349\tRice\tTX\tNavarro County\tH1\n75933\t48351\tCall\tTX\tNewton County\tH1\n77632\t48351\tOrange\tTX\tNewton County\tH1\n75928\t48351\tBon wier\tTX\tNewton County\tH1\n75966\t48351\tNewton\tTX\tNewton County\tH1\n75951\t48351\tJasper\tTX\tNewton County\tH1\n75956\t48351\tKirbyville\tTX\tNewton County\tH1\n75932\t48351\tBurkeville\tTX\tNewton County\tH1\n75977\t48351\tWiergate\tTX\tNewton County\tH1\n77614\t48351\tDeweyville\tTX\tNewton County\tH1\n77612\t48351\tBuna\tTX\tNewton County\tH1\n79532\t48353\tLoraine\tTX\tNolan County\tH1\n79545\t48353\tRoscoe\tTX\tNolan County\tH1\n79506\t48353\tBlackwell\tTX\tNolan County\tH1\n79537\t48353\tNolan\tTX\tNolan County\tH1\n79535\t48353\tMaryneal\tTX\tNolan County\tH1\n79556\t48353\tSweetwater\tTX\tNolan County\tH1\n78418\t48355\tCorpus christi\tTX\tNueces County\tH1\n78401\t48355\tCorpus christi\tTX\tNueces County\tH1\n78466\t48355\tCorpus christi\tTX\tNueces County\tH1\n78383\t48355\tSandia\tTX\tNueces County\tH1\n78410\t48355\tCorpus christi\tTX\tNueces County\tH1\n78412\t48355\tCorpus christi\tTX\tNueces County\tH1\n78407\t48355\tCorpus christi\tTX\tNueces County\tH1\n78467\t48355\tCorpus christi\tTX\tNueces County\tH1\n78463\t48355\tCorpus christi\tTX\tNueces County\tH1\n78404\t48355\tCorpus christi\tTX\tNueces County\tH1\n78413\t48355\tCorpus christi\tTX\tNueces County\tH1\n78406\t48355\tCorpus christi\tTX\tNueces County\tH1\n78403\t48355\tCorpus christi\tTX\tNueces County\tH1\n78480\t48355\tCorpus christi\tTX\tNueces County\tH1\n78351\t48355\tDriscoll\tTX\tNueces County\tH1\n78363\t48355\tKingsville\tTX\tNueces County\tH1\n78405\t48355\tCorpus christi\tTX\tNueces County\tH1\n78460\t48355\tCorpus christi\tTX\tNueces County\tH1\n78408\t48355\tCorpus christi\tTX\tNueces County\tH1\n78339\t48355\tBanquete\tTX\tNueces County\tH1\n78380\t48355\tRobstown\tTX\tNueces County\tH1\n78411\t48355\tCorpus christi\tTX\tNueces County\tH1\n78426\t48355\tCorpus christi\tTX\tNueces County\tH1\n78419\t48355\tCorpus christi\tTX\tNueces County\tH1\n78347\t48355\tChapman ranch\tTX\tNueces County\tH1\n78330\t48355\tAgua dulce\tTX\tNueces County\tH1\n78402\t48355\tCorpus christi\tTX\tNueces County\tH1\n78465\t48355\tCorpus christi\tTX\tNueces County\tH1\n78336\t48355\tAransas pass\tTX\tNueces County\tH1\n78373\t48355\tPort aransas\tTX\tNueces County\tH1\n78343\t48355\tBishop\tTX\tNueces County\tH1\n78415\t48355\tCorpus christi\tTX\tNueces County\tH1\n78417\t48355\tCorpus christi\tTX\tNueces County\tH1\n78414\t48355\tCorpus christi\tTX\tNueces County\tH1\n78468\t48355\tCorpus christi\tTX\tNueces County\tH1\n78469\t48355\tCorpus christi\tTX\tNueces County\tH1\n78427\t48355\tCorpus christi\tTX\tNueces County\tH1\n78416\t48355\tCorpus christi\tTX\tNueces County\tH1\n78409\t48355\tCorpus christi\tTX\tNueces County\tH1\n79070\t48357\tPerryton\tTX\tOchiltree County\tH1\n79033\t48357\tFarnsworth\tTX\tOchiltree County\tH1\n79093\t48357\tWaka\tTX\tOchiltree County\tH1\n79098\t48359\tWildorado\tTX\tOldham County\tH1\n79092\t48359\tVega\tTX\tOldham County\tH1\n79001\t48359\tAdrian\tTX\tOldham County\tH1\n79010\t48359\tBoys ranch\tTX\tOldham County\tH1\n77632\t48361\tOrange\tTX\tOrange County\tH1\n77611\t48361\tBridge city\tTX\tOrange County\tH1\n77639\t48361\tOrangefield\tTX\tOrange County\tH1\n77662\t48361\tVidor\tTX\tOrange County\tH1\n77630\t48361\tOrange\tTX\tOrange County\tH1\n77670\t48361\tVidor\tTX\tOrange County\tH1\n77626\t48361\tMauriceville\tTX\tOrange County\tH1\n76449\t48363\tGraford\tTX\tPalo Pinto County\tH1\n76067\t48363\tMineral wells\tTX\tPalo Pinto County\tH1\n76462\t48363\tLipan\tTX\tPalo Pinto County\tH1\n76429\t48363\tCaddo\tTX\tPalo Pinto County\tH1\n76453\t48363\tGordon\tTX\tPalo Pinto County\tH1\n76486\t48363\tPerrin\tTX\tPalo Pinto County\tH1\n76066\t48363\tMillsap\tTX\tPalo Pinto County\tH1\n76472\t48363\tSanto\tTX\tPalo Pinto County\tH1\n76475\t48363\tStrawn\tTX\tPalo Pinto County\tH1\n76484\t48363\tPalo pinto\tTX\tPalo Pinto County\tH1\n76463\t48363\tMingus\tTX\tPalo Pinto County\tH1\n76450\t48363\tGraham\tTX\tPalo Pinto County\tH1\n75639\t48365\tDe berry\tTX\tPanola County\tH1\n75669\t48365\tLong branch\tTX\tPanola County\tH1\n75652\t48365\tHenderson\tTX\tPanola County\tH1\n75975\t48365\tTimpson\tTX\tPanola County\tH1\n75672\t48365\tMarshall\tTX\tPanola County\tH1\n75685\t48365\tPanola\tTX\tPanola County\tH1\n75974\t48365\tTenaha\tTX\tPanola County\tH1\n75692\t48365\tWaskom\tTX\tPanola County\tH1\n75691\t48365\tTatum\tTX\tPanola County\tH1\n75637\t48365\tClayton\tTX\tPanola County\tH1\n75633\t48365\tCarthage\tTX\tPanola County\tH1\n75643\t48365\tGary\tTX\tPanola County\tH1\n75631\t48365\tBeckville\tTX\tPanola County\tH1\n75954\t48365\tJoaquin\tTX\tPanola County\tH1\n76085\t48367\tWeatherford\tTX\tParker County\tH1\n76035\t48367\tCresson\tTX\tParker County\tH1\n76067\t48367\tMineral wells\tTX\tParker County\tH1\n76086\t48367\tWeatherford\tTX\tParker County\tH1\n76108\t48367\tFort worth\tTX\tParker County\tH1\n76462\t48367\tLipan\tTX\tParker County\tH1\n76485\t48367\tPeaster\tTX\tParker County\tH1\n76088\t48367\tWeatherford\tTX\tParker County\tH1\n76020\t48367\tAzle\tTX\tParker County\tH1\n76487\t48367\tPoolville\tTX\tParker County\tH1\n76486\t48367\tPerrin\tTX\tParker County\tH1\n76049\t48367\tGranbury\tTX\tParker County\tH1\n76023\t48367\tBoyd\tTX\tParker County\tH1\n76066\t48367\tMillsap\tTX\tParker County\tH1\n76082\t48367\tSpringtown\tTX\tParker County\tH1\n76490\t48367\tWhitt\tTX\tParker County\tH1\n76439\t48367\tDennis\tTX\tParker County\tH1\n76087\t48367\tWeatherford\tTX\tParker County\tH1\n76098\t48367\tAzle\tTX\tParker County\tH1\n76126\t48367\tFort worth\tTX\tParker County\tH1
